vi "Convert TDMS channel.vi"(1 "dt":dbl=nan, 2 "End time":dbl=nan, 4 "Start time":dbl=nan, 6 "buffer size (-1: all)":i64=100000 format="%.0p", 7 "Output tdms ref":refnum<k34>, 8 "Error In":errorcluster, 9 "Channel name":string, 10 "Group name":string, 11 "Input tdms ref":refnum<k34>) -> (0 "Error Out":errorcluster, 3 "Input tdms ref out":refnum<k34>, 5 "Output tdms ref out":refnum<k34>)   [LabVIEW 2016]
uses:
  Utilities/Replace dt DBL.vi
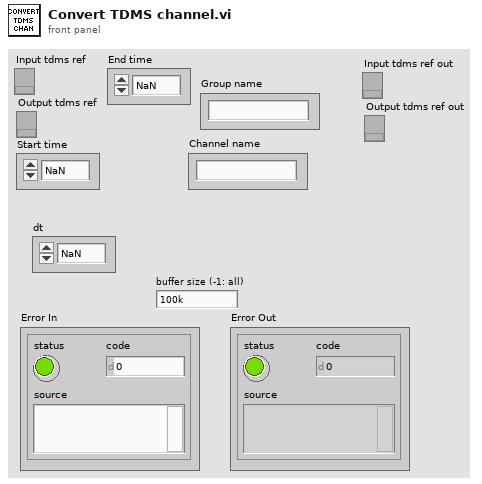
[diagram p1: front panel]
types:
  T1 = typedef "TDMS channel info.ctl" = cluster{"t0":timestamp, "dt":dbl, "Channel length":i64}
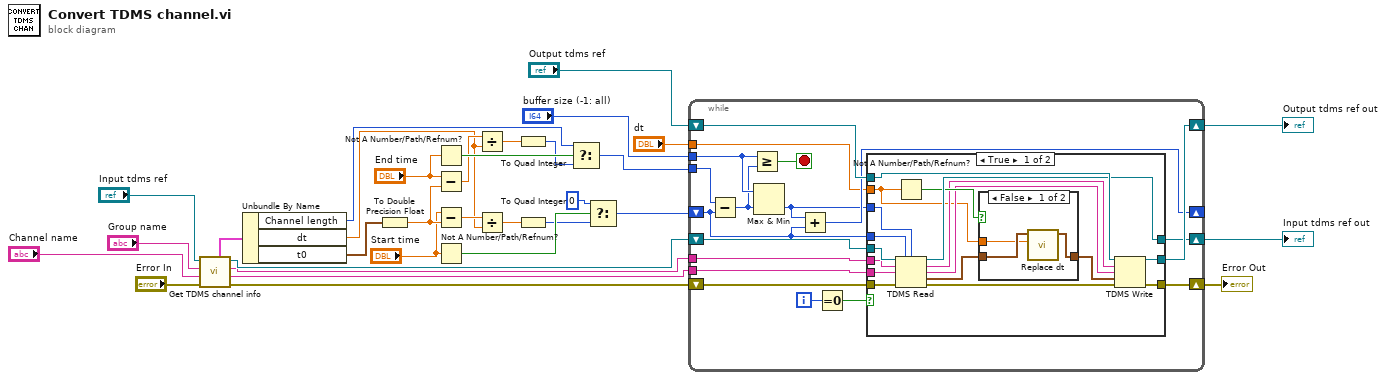
[diagram p0: block diagram]
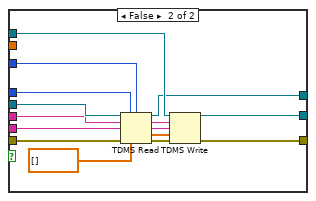
[diagram p3: hidden frame]
diagram:
  n1 = call "Get TDMS channel info.vi"("error in"="Error In", "Channel name"="Channel name", "group name"="Group name", "tdms file"="Input tdms ref") -> ("error out"=w7:errorcluster, "channel name out"=w1:string, "group name out"=w3:string, "tdms file out"=w8:refnum<k34>, "TDMS channel info"=w10:T1)  [unwired: 3 in]
  n2 = Unbundle By Name(w10) -> ("Channel length"=w6:i64, "dt"=w9:dbl, "t0"=w5:timestamp)
  n3 = To Double Precision Float(number=w5) -> (double precision float=w16:dbl)
  n4 = Not A Number/Path/Refnum?(number/path/refnum="End time") -> (NaN/Path/Refnum?=w27:bool)
  n5 = Subtract(x="End time", y=w16) -> (x-y=w26:dbl)
  n6 = Subtract(x="Start time", y=w16) -> (x-y=w30:dbl)
  n7 = Not A Number/Path/Refnum?(number/path/refnum="Start time") -> (NaN/Path/Refnum?=w32:bool)
  n8 = Divide(x=w26, y=w9) -> (x/y=w24:dbl)
  n9 = Divide(x=w30, y=w9) -> (x/y=w29:dbl)
  n10 = To Quad Integer(1:w24) -> (0:w25:i64)
  n11 = To Quad Integer(1:w29) -> (0:w28:i64)
  n12 = Select(t=w6, s=w27, f=w25) -> (s? t:f=w20:i64)
  n13 = Select(t=i64 0 ("offset (0)"), s=w32, f=w28) -> (s? t:f=w22:i64)
  n14 = while {
    tunnel: w3 -> [w46]
    tunnel: w1 -> [w45]
    shift-right: [w39] -> w18
    shift-left: w8 -> [w50]
    shift-right: [w44] -> w17
    shift-left: w7 -> [w49]
    tunnel: "buffer size (-1: all)" -> [w42]
    shift-right: [w38] -> _
    shift-left: w22 -> [w33]
    shift-right: [w47] -> w19
    shift-left: "Output tdms ref" -> [w48]
    tunnel: w20 -> [w43]
    tunnel: "dt" -> [w35]
    i -> [w37]
    stop <- w40 stop-if-true
    n15 = Subtract(x=w43, y=w33) -> (x-y=w41:i64)
    n16 = Greater Or Equal?(x=w42, y=w41) -> (x >= y?=w40:bool)
    n17 = Max & Min(x=w42, y=w41) -> (min(x,y)=w34:i64)  [unwired: 1 out]
    n18 = Add(x=w34, y=w33) -> (x+y=w38:i64)
    n19 = Equal To 0?(x=w37) -> (x = 0?=w36:bool)
    n20 = case shown="True" w36 {
      tunnel: w50 -> [w67 w86]
      tunnel: w49 -> [w66 w85]
      tunnel: w48 -> [w64 w83]
      tunnel: [w63 w82] -> w47
      tunnel: w46 -> [w62 w73]
      tunnel: w45 -> [w54 w76]
      tunnel: [w61 w81] -> w44
      tunnel: [w60 w80] -> w39
      tunnel: w33 -> [w58 w79]
      tunnel: w34 -> [w57 w78]
      tunnel: w35 -> [w51 _]
      frame True {
        n21 = Not A Number/Path/Refnum?(number/path/refnum=w51) -> (NaN/Path/Refnum?=w55:bool)
        n22 = TDMS Read(0:w67, 1:w58, 2:w57, 5:w62, 7:w54, 11:w66) -> (4:w60:refnum<k34>, 6:w52:string, 8:w53:string, 10:w59:waveform(dbl), 15:w65:errorcluster)  [unwired: 2 in, 1 out]
        n23 = case shown="False" w55 {
          tunnel: w59 -> [w69 w71]
          tunnel: [w70 w71] -> w56
          tunnel: w51 -> [w68 _]
          frame False {
            n24 = call-poly "Replace dt.vi"("dt"=w68, "Waveform in"=w69) -> ("Waveform out"=w70:waveform(dbl))  [unwired: 9 in]
          }
          frame True {
          }
        }
        n25 = TDMS Write(0:w64, 5:w52, 7:w53, 9:w56, 11:w65) -> (4:w63:refnum<k34>, 15:w61:errorcluster)  [unwired: 1 in, 2 out]
      }
      frame False {
        n26 = TDMS Read(0:w86, 1:w79, 2:w78, 5:w73, 7:w76, 11:w85, 12:dbl[] []) -> (4:w80:refnum<k34>, 6:w72:string, 8:w75:string, 10:w74:dbl[], 15:w84:errorcluster)  [unwired: 1 in, 1 out]
        n27 = TDMS Write(0:w83, 5:w72, 7:w75, 9:w74, 11:w84) -> (4:w82:refnum<k34>, 15:w81:errorcluster)  [unwired: 1 in, 2 out]
      }
    }
  }
  "Input tdms ref out" <- w18
  "Output tdms ref out" <- w19
  "Error Out" <- w17
